vi "matrix_transpose_empty.vi"   [LabVIEW 2020]
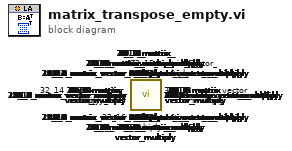
[diagram p0: block diagram]
diagram:
  n1 = call <vilib>:"32_16_matrix_vector_multiply.vi"() -> ()  [unwired: 6 in, 1 out]
  n2 = call <vilib>:"32_15_matrix_vector_multiply.vi"() -> ()  [unwired: 6 in, 1 out]
  n3 = call <vilib>:"32_14_matrix_vector_multiply.vi"() -> ()  [unwired: 6 in, 1 out]
  n4 = call <vilib>:"32_13_matrix_vector_multiply.vi"() -> ()  [unwired: 6 in, 1 out]
  n5 = call <vilib>:"32_12_matrix_vector_multiply.vi"() -> ()  [unwired: 6 in, 1 out]
  n6 = call <vilib>:"32_11_matrix_vector_multiply.vi"() -> ()  [unwired: 6 in, 1 out]
  n7 = call <vilib>:"32_10_matrix_vector_multiply.vi"() -> ()  [unwired: 6 in, 1 out]
  n8 = call <vilib>:"32_9_matrix_vector_multiply.vi"() -> ()  [unwired: 6 in, 1 out]
  n9 = call <vilib>:"32_8_matrix_vector_multiply.vi"() -> ()  [unwired: 6 in, 1 out]
  n10 = call <vilib>:"32_7_matrix_vector_multiply.vi"() -> ()  [unwired: 6 in, 1 out]
  n11 = call <vilib>:"32_6_matrix_vector_multiply.vi"() -> ()  [unwired: 6 in, 1 out]
  n12 = call <vilib>:"32_5_matrix_vector_multiply.vi"() -> ()  [unwired: 6 in, 1 out]
  n13 = call <vilib>:"32_4_matrix_vector_multiply.vi"() -> ()  [unwired: 6 in, 1 out]
  n14 = call <vilib>:"32_3_matrix_vector_multiply.vi"() -> ()  [unwired: 6 in, 1 out]
  n15 = call <vilib>:"32_2_matrix_vector_multiply.vi"() -> ()  [unwired: 6 in, 1 out]
  n16 = call <vilib>:"32_1_matrix_vector_multiply.vi"() -> ()  [unwired: 6 in, 1 out]
  n17 = call <vilib>:"31_16_matrix_vector_multiply.vi"() -> ()  [unwired: 6 in, 1 out]
  n18 = call <vilib>:"31_15_matrix_vector_multiply.vi"() -> ()  [unwired: 6 in, 1 out]
  n19 = call <vilib>:"31_14_matrix_vector_multiply.vi"() -> ()  [unwired: 6 in, 1 out]
  n20 = call <vilib>:"31_13_matrix_vector_multiply.vi"() -> ()  [unwired: 6 in, 1 out]
  n21 = call <vilib>:"31_12_matrix_vector_multiply.vi"() -> ()  [unwired: 6 in, 1 out]
  n22 = call <vilib>:"31_11_matrix_vector_multiply.vi"() -> ()  [unwired: 6 in, 1 out]
  n23 = call <vilib>:"31_10_matrix_vector_multiply.vi"() -> ()  [unwired: 6 in, 1 out]
  n24 = call <vilib>:"31_9_matrix_vector_multiply.vi"() -> ()  [unwired: 6 in, 1 out]
  n25 = call <vilib>:"31_8_matrix_vector_multiply.vi"() -> ()  [unwired: 6 in, 1 out]
  n26 = call <vilib>:"31_7_matrix_vector_multiply.vi"() -> ()  [unwired: 6 in, 1 out]
  n27 = call <vilib>:"31_6_matrix_vector_multiply.vi"() -> ()  [unwired: 6 in, 1 out]
  n28 = call <vilib>:"31_5_matrix_vector_multiply.vi"() -> ()  [unwired: 6 in, 1 out]
  n29 = call <vilib>:"31_4_matrix_vector_multiply.vi"() -> ()  [unwired: 6 in, 1 out]
  n30 = call <vilib>:"31_3_matrix_vector_multiply.vi"() -> ()  [unwired: 6 in, 1 out]
  n31 = call <vilib>:"31_2_matrix_vector_multiply.vi"() -> ()  [unwired: 6 in, 1 out]
  n32 = call <vilib>:"31_1_matrix_vector_multiply.vi"() -> ()  [unwired: 6 in, 1 out]
  n33 = call <vilib>:"30_16_matrix_vector_multiply.vi"() -> ()  [unwired: 6 in, 1 out]
  n34 = call <vilib>:"30_15_matrix_vector_multiply.vi"() -> ()  [unwired: 6 in, 1 out]
  n35 = call <vilib>:"30_14_matrix_vector_multiply.vi"() -> ()  [unwired: 6 in, 1 out]
  n36 = call <vilib>:"30_13_matrix_vector_multiply.vi"() -> ()  [unwired: 6 in, 1 out]
  n37 = call <vilib>:"30_12_matrix_vector_multiply.vi"() -> ()  [unwired: 6 in, 1 out]
  n38 = call <vilib>:"30_11_matrix_vector_multiply.vi"() -> ()  [unwired: 6 in, 1 out]
  n39 = call <vilib>:"30_10_matrix_vector_multiply.vi"() -> ()  [unwired: 6 in, 1 out]
  n40 = call <vilib>:"30_9_matrix_vector_multiply.vi"() -> ()  [unwired: 6 in, 1 out]
  n41 = call <vilib>:"30_8_matrix_vector_multiply.vi"() -> ()  [unwired: 6 in, 1 out]
  n42 = call <vilib>:"30_7_matrix_vector_multiply.vi"() -> ()  [unwired: 6 in, 1 out]
  n43 = call <vilib>:"30_6_matrix_vector_multiply.vi"() -> ()  [unwired: 6 in, 1 out]
  n44 = call <vilib>:"30_5_matrix_vector_multiply.vi"() -> ()  [unwired: 6 in, 1 out]
  n45 = call <vilib>:"30_4_matrix_vector_multiply.vi"() -> ()  [unwired: 6 in, 1 out]
  n46 = call <vilib>:"30_3_matrix_vector_multiply.vi"() -> ()  [unwired: 6 in, 1 out]
  n47 = call <vilib>:"30_2_matrix_vector_multiply.vi"() -> ()  [unwired: 6 in, 1 out]
  n48 = call <vilib>:"30_1_matrix_vector_multiply.vi"() -> ()  [unwired: 6 in, 1 out]
  n49 = call <vilib>:"29_16_matrix_vector_multiply.vi"() -> ()  [unwired: 6 in, 1 out]
  n50 = call <vilib>:"29_15_matrix_vector_multiply.vi"() -> ()  [unwired: 6 in, 1 out]
  n51 = call <vilib>:"29_14_matrix_vector_multiply.vi"() -> ()  [unwired: 6 in, 1 out]
  n52 = call <vilib>:"29_13_matrix_vector_multiply.vi"() -> ()  [unwired: 6 in, 1 out]
  n53 = call <vilib>:"29_12_matrix_vector_multiply.vi"() -> ()  [unwired: 6 in, 1 out]
  n54 = call <vilib>:"29_11_matrix_vector_multiply.vi"() -> ()  [unwired: 6 in, 1 out]
  n55 = call <vilib>:"29_10_matrix_vector_multiply.vi"() -> ()  [unwired: 6 in, 1 out]
  n56 = call <vilib>:"29_9_matrix_vector_multiply.vi"() -> ()  [unwired: 6 in, 1 out]
  n57 = call <vilib>:"29_8_matrix_vector_multiply.vi"() -> ()  [unwired: 6 in, 1 out]
  n58 = call <vilib>:"29_7_matrix_vector_multiply.vi"() -> ()  [unwired: 6 in, 1 out]
  n59 = call <vilib>:"29_6_matrix_vector_multiply.vi"() -> ()  [unwired: 6 in, 1 out]
  n60 = call <vilib>:"29_5_matrix_vector_multiply.vi"() -> ()  [unwired: 6 in, 1 out]
  n61 = call <vilib>:"29_4_matrix_vector_multiply.vi"() -> ()  [unwired: 6 in, 1 out]
  n62 = call <vilib>:"29_3_matrix_vector_multiply.vi"() -> ()  [unwired: 6 in, 1 out]
  n63 = call <vilib>:"29_2_matrix_vector_multiply.vi"() -> ()  [unwired: 6 in, 1 out]
  n64 = call <vilib>:"29_1_matrix_vector_multiply.vi"() -> ()  [unwired: 6 in, 1 out]
  n65 = call <vilib>:"28_16_matrix_vector_multiply.vi"() -> ()  [unwired: 6 in, 1 out]
  n66 = call <vilib>:"28_15_matrix_vector_multiply.vi"() -> ()  [unwired: 6 in, 1 out]
  n67 = call <vilib>:"28_14_matrix_vector_multiply.vi"() -> ()  [unwired: 6 in, 1 out]
  n68 = call <vilib>:"28_13_matrix_vector_multiply.vi"() -> ()  [unwired: 6 in, 1 out]
  n69 = call <vilib>:"28_12_matrix_vector_multiply.vi"() -> ()  [unwired: 6 in, 1 out]
  n70 = call <vilib>:"28_11_matrix_vector_multiply.vi"() -> ()  [unwired: 6 in, 1 out]
  n71 = call <vilib>:"28_10_matrix_vector_multiply.vi"() -> ()  [unwired: 6 in, 1 out]
  n72 = call <vilib>:"28_9_matrix_vector_multiply.vi"() -> ()  [unwired: 6 in, 1 out]
  n73 = call <vilib>:"28_8_matrix_vector_multiply.vi"() -> ()  [unwired: 6 in, 1 out]
  n74 = call <vilib>:"28_7_matrix_vector_multiply.vi"() -> ()  [unwired: 6 in, 1 out]
  n75 = call <vilib>:"28_6_matrix_vector_multiply.vi"() -> ()  [unwired: 6 in, 1 out]
  n76 = call <vilib>:"28_5_matrix_vector_multiply.vi"() -> ()  [unwired: 6 in, 1 out]
  n77 = call <vilib>:"28_4_matrix_vector_multiply.vi"() -> ()  [unwired: 6 in, 1 out]
  n78 = call <vilib>:"28_3_matrix_vector_multiply.vi"() -> ()  [unwired: 6 in, 1 out]
  n79 = call <vilib>:"28_2_matrix_vector_multiply.vi"() -> ()  [unwired: 6 in, 1 out]
  n80 = call <vilib>:"28_1_matrix_vector_multiply.vi"() -> ()  [unwired: 6 in, 1 out]
  n81 = call <vilib>:"27_16_matrix_vector_multiply.vi"() -> ()  [unwired: 6 in, 1 out]
  n82 = call <vilib>:"27_15_matrix_vector_multiply.vi"() -> ()  [unwired: 6 in, 1 out]
  n83 = call <vilib>:"27_14_matrix_vector_multiply.vi"() -> ()  [unwired: 6 in, 1 out]
  n84 = call <vilib>:"27_13_matrix_vector_multiply.vi"() -> ()  [unwired: 6 in, 1 out]
  n85 = call <vilib>:"27_12_matrix_vector_multiply.vi"() -> ()  [unwired: 6 in, 1 out]
  n86 = call <vilib>:"27_11_matrix_vector_multiply.vi"() -> ()  [unwired: 6 in, 1 out]
  n87 = call <vilib>:"27_10_matrix_vector_multiply.vi"() -> ()  [unwired: 6 in, 1 out]
  n88 = call <vilib>:"27_9_matrix_vector_multiply.vi"() -> ()  [unwired: 6 in, 1 out]
  n89 = call <vilib>:"27_8_matrix_vector_multiply.vi"() -> ()  [unwired: 6 in, 1 out]
  n90 = call <vilib>:"27_7_matrix_vector_multiply.vi"() -> ()  [unwired: 6 in, 1 out]
  n91 = call <vilib>:"27_6_matrix_vector_multiply.vi"() -> ()  [unwired: 6 in, 1 out]
  n92 = call <vilib>:"27_5_matrix_vector_multiply.vi"() -> ()  [unwired: 6 in, 1 out]
  n93 = call <vilib>:"27_4_matrix_vector_multiply.vi"() -> ()  [unwired: 6 in, 1 out]
  n94 = call <vilib>:"27_3_matrix_vector_multiply.vi"() -> ()  [unwired: 6 in, 1 out]
  n95 = call <vilib>:"27_2_matrix_vector_multiply.vi"() -> ()  [unwired: 6 in, 1 out]
  n96 = call <vilib>:"27_1_matrix_vector_multiply.vi"() -> ()  [unwired: 6 in, 1 out]
  n97 = call <vilib>:"26_16_matrix_vector_multiply.vi"() -> ()  [unwired: 6 in, 1 out]
  n98 = call <vilib>:"26_15_matrix_vector_multiply.vi"() -> ()  [unwired: 6 in, 1 out]
  n99 = call <vilib>:"26_14_matrix_vector_multiply.vi"() -> ()  [unwired: 6 in, 1 out]
  n100 = call <vilib>:"26_13_matrix_vector_multiply.vi"() -> ()  [unwired: 6 in, 1 out]
  n101 = call <vilib>:"26_12_matrix_vector_multiply.vi"() -> ()  [unwired: 6 in, 1 out]
  n102 = call <vilib>:"26_11_matrix_vector_multiply.vi"() -> ()  [unwired: 6 in, 1 out]
  n103 = call <vilib>:"26_10_matrix_vector_multiply.vi"() -> ()  [unwired: 6 in, 1 out]
  n104 = call <vilib>:"26_9_matrix_vector_multiply.vi"() -> ()  [unwired: 6 in, 1 out]
  n105 = call <vilib>:"26_8_matrix_vector_multiply.vi"() -> ()  [unwired: 6 in, 1 out]
  n106 = call <vilib>:"26_7_matrix_vector_multiply.vi"() -> ()  [unwired: 6 in, 1 out]
  n107 = call <vilib>:"26_6_matrix_vector_multiply.vi"() -> ()  [unwired: 6 in, 1 out]
  n108 = call <vilib>:"26_5_matrix_vector_multiply.vi"() -> ()  [unwired: 6 in, 1 out]
  n109 = call <vilib>:"26_4_matrix_vector_multiply.vi"() -> ()  [unwired: 6 in, 1 out]
  n110 = call <vilib>:"26_3_matrix_vector_multiply.vi"() -> ()  [unwired: 6 in, 1 out]
  n111 = call <vilib>:"26_2_matrix_vector_multiply.vi"() -> ()  [unwired: 6 in, 1 out]
  n112 = call <vilib>:"26_1_matrix_vector_multiply.vi"() -> ()  [unwired: 6 in, 1 out]
  n113 = call <vilib>:"25_16_matrix_vector_multiply.vi"() -> ()  [unwired: 6 in, 1 out]
  n114 = call <vilib>:"25_15_matrix_vector_multiply.vi"() -> ()  [unwired: 6 in, 1 out]
  n115 = call <vilib>:"25_14_matrix_vector_multiply.vi"() -> ()  [unwired: 6 in, 1 out]
  n116 = call <vilib>:"25_13_matrix_vector_multiply.vi"() -> ()  [unwired: 6 in, 1 out]
  n117 = call <vilib>:"25_12_matrix_vector_multiply.vi"() -> ()  [unwired: 6 in, 1 out]
  n118 = call <vilib>:"25_11_matrix_vector_multiply.vi"() -> ()  [unwired: 6 in, 1 out]
  n119 = call <vilib>:"25_10_matrix_vector_multiply.vi"() -> ()  [unwired: 6 in, 1 out]
  n120 = call <vilib>:"25_9_matrix_vector_multiply.vi"() -> ()  [unwired: 6 in, 1 out]
  n121 = call <vilib>:"25_8_matrix_vector_multiply.vi"() -> ()  [unwired: 6 in, 1 out]
  n122 = call <vilib>:"25_7_matrix_vector_multiply.vi"() -> ()  [unwired: 6 in, 1 out]
  n123 = call <vilib>:"25_6_matrix_vector_multiply.vi"() -> ()  [unwired: 6 in, 1 out]
  n124 = call <vilib>:"25_5_matrix_vector_multiply.vi"() -> ()  [unwired: 6 in, 1 out]
  n125 = call <vilib>:"25_4_matrix_vector_multiply.vi"() -> ()  [unwired: 6 in, 1 out]
  n126 = call <vilib>:"25_3_matrix_vector_multiply.vi"() -> ()  [unwired: 6 in, 1 out]
  n127 = call <vilib>:"25_2_matrix_vector_multiply.vi"() -> ()  [unwired: 6 in, 1 out]
  n128 = call <vilib>:"25_1_matrix_vector_multiply.vi"() -> ()  [unwired: 6 in, 1 out]
  n129 = call <vilib>:"24_16_matrix_vector_multiply.vi"() -> ()  [unwired: 6 in, 1 out]
  n130 = call <vilib>:"24_15_matrix_vector_multiply.vi"() -> ()  [unwired: 6 in, 1 out]
  n131 = call <vilib>:"24_14_matrix_vector_multiply.vi"() -> ()  [unwired: 6 in, 1 out]
  n132 = call <vilib>:"24_13_matrix_vector_multiply.vi"() -> ()  [unwired: 6 in, 1 out]
  n133 = call <vilib>:"24_12_matrix_vector_multiply.vi"() -> ()  [unwired: 6 in, 1 out]
  n134 = call <vilib>:"24_11_matrix_vector_multiply.vi"() -> ()  [unwired: 6 in, 1 out]
  n135 = call <vilib>:"24_10_matrix_vector_multiply.vi"() -> ()  [unwired: 6 in, 1 out]
  n136 = call <vilib>:"24_9_matrix_vector_multiply.vi"() -> ()  [unwired: 6 in, 1 out]
  n137 = call <vilib>:"24_8_matrix_vector_multiply.vi"() -> ()  [unwired: 6 in, 1 out]
  n138 = call <vilib>:"24_7_matrix_vector_multiply.vi"() -> ()  [unwired: 6 in, 1 out]
  n139 = call <vilib>:"24_6_matrix_vector_multiply.vi"() -> ()  [unwired: 6 in, 1 out]
  n140 = call <vilib>:"24_5_matrix_vector_multiply.vi"() -> ()  [unwired: 6 in, 1 out]
  n141 = call <vilib>:"24_4_matrix_vector_multiply.vi"() -> ()  [unwired: 6 in, 1 out]
  n142 = call <vilib>:"24_3_matrix_vector_multiply.vi"() -> ()  [unwired: 6 in, 1 out]
  n143 = call <vilib>:"24_2_matrix_vector_multiply.vi"() -> ()  [unwired: 6 in, 1 out]
  n144 = call <vilib>:"24_1_matrix_vector_multiply.vi"() -> ()  [unwired: 6 in, 1 out]
  n145 = call <vilib>:"23_16_matrix_vector_multiply.vi"() -> ()  [unwired: 6 in, 1 out]
  n146 = call <vilib>:"23_15_matrix_vector_multiply.vi"() -> ()  [unwired: 6 in, 1 out]
  n147 = call <vilib>:"23_14_matrix_vector_multiply.vi"() -> ()  [unwired: 6 in, 1 out]
  n148 = call <vilib>:"23_13_matrix_vector_multiply.vi"() -> ()  [unwired: 6 in, 1 out]
  n149 = call <vilib>:"23_12_matrix_vector_multiply.vi"() -> ()  [unwired: 6 in, 1 out]
  n150 = call <vilib>:"23_11_matrix_vector_multiply.vi"() -> ()  [unwired: 6 in, 1 out]
  n151 = call <vilib>:"23_10_matrix_vector_multiply.vi"() -> ()  [unwired: 6 in, 1 out]
  n152 = call <vilib>:"23_9_matrix_vector_multiply.vi"() -> ()  [unwired: 6 in, 1 out]
  n153 = call <vilib>:"23_8_matrix_vector_multiply.vi"() -> ()  [unwired: 6 in, 1 out]
  n154 = call <vilib>:"23_7_matrix_vector_multiply.vi"() -> ()  [unwired: 6 in, 1 out]
  n155 = call <vilib>:"23_6_matrix_vector_multiply.vi"() -> ()  [unwired: 6 in, 1 out]
  n156 = call <vilib>:"23_5_matrix_vector_multiply.vi"() -> ()  [unwired: 6 in, 1 out]
  n157 = call <vilib>:"23_4_matrix_vector_multiply.vi"() -> ()  [unwired: 6 in, 1 out]
  n158 = call <vilib>:"23_3_matrix_vector_multiply.vi"() -> ()  [unwired: 6 in, 1 out]
  n159 = call <vilib>:"23_2_matrix_vector_multiply.vi"() -> ()  [unwired: 6 in, 1 out]
  n160 = call <vilib>:"23_1_matrix_vector_multiply.vi"() -> ()  [unwired: 6 in, 1 out]
  n161 = call <vilib>:"22_16_matrix_vector_multiply.vi"() -> ()  [unwired: 6 in, 1 out]
  n162 = call <vilib>:"22_15_matrix_vector_multiply.vi"() -> ()  [unwired: 6 in, 1 out]
  n163 = call <vilib>:"22_14_matrix_vector_multiply.vi"() -> ()  [unwired: 6 in, 1 out]
  n164 = call <vilib>:"22_13_matrix_vector_multiply.vi"() -> ()  [unwired: 6 in, 1 out]
  n165 = call <vilib>:"22_12_matrix_vector_multiply.vi"() -> ()  [unwired: 6 in, 1 out]
  n166 = call <vilib>:"22_11_matrix_vector_multiply.vi"() -> ()  [unwired: 6 in, 1 out]
  n167 = call <vilib>:"22_10_matrix_vector_multiply.vi"() -> ()  [unwired: 6 in, 1 out]
  n168 = call <vilib>:"22_9_matrix_vector_multiply.vi"() -> ()  [unwired: 6 in, 1 out]
  n169 = call <vilib>:"22_8_matrix_vector_multiply.vi"() -> ()  [unwired: 6 in, 1 out]
  n170 = call <vilib>:"22_7_matrix_vector_multiply.vi"() -> ()  [unwired: 6 in, 1 out]
  n171 = call <vilib>:"22_6_matrix_vector_multiply.vi"() -> ()  [unwired: 6 in, 1 out]
  n172 = call <vilib>:"22_5_matrix_vector_multiply.vi"() -> ()  [unwired: 6 in, 1 out]
  n173 = call <vilib>:"22_4_matrix_vector_multiply.vi"() -> ()  [unwired: 6 in, 1 out]
  n174 = call <vilib>:"22_3_matrix_vector_multiply.vi"() -> ()  [unwired: 6 in, 1 out]
  n175 = call <vilib>:"22_2_matrix_vector_multiply.vi"() -> ()  [unwired: 6 in, 1 out]
  n176 = call <vilib>:"22_1_matrix_vector_multiply.vi"() -> ()  [unwired: 6 in, 1 out]
  n177 = call <vilib>:"21_16_matrix_vector_multiply.vi"() -> ()  [unwired: 6 in, 1 out]
  n178 = call <vilib>:"21_15_matrix_vector_multiply.vi"() -> ()  [unwired: 6 in, 1 out]
  n179 = call <vilib>:"21_14_matrix_vector_multiply.vi"() -> ()  [unwired: 6 in, 1 out]
  n180 = call <vilib>:"21_13_matrix_vector_multiply.vi"() -> ()  [unwired: 6 in, 1 out]
  n181 = call <vilib>:"21_12_matrix_vector_multiply.vi"() -> ()  [unwired: 6 in, 1 out]
  n182 = call <vilib>:"21_11_matrix_vector_multiply.vi"() -> ()  [unwired: 6 in, 1 out]
  n183 = call <vilib>:"21_10_matrix_vector_multiply.vi"() -> ()  [unwired: 6 in, 1 out]
  n184 = call <vilib>:"21_9_matrix_vector_multiply.vi"() -> ()  [unwired: 6 in, 1 out]
  n185 = call <vilib>:"21_8_matrix_vector_multiply.vi"() -> ()  [unwired: 6 in, 1 out]
  n186 = call <vilib>:"21_7_matrix_vector_multiply.vi"() -> ()  [unwired: 6 in, 1 out]
  n187 = call <vilib>:"21_6_matrix_vector_multiply.vi"() -> ()  [unwired: 6 in, 1 out]
  n188 = call <vilib>:"21_5_matrix_vector_multiply.vi"() -> ()  [unwired: 6 in, 1 out]
  n189 = call <vilib>:"21_4_matrix_vector_multiply.vi"() -> ()  [unwired: 6 in, 1 out]
  n190 = call <vilib>:"21_3_matrix_vector_multiply.vi"() -> ()  [unwired: 6 in, 1 out]
  n191 = call <vilib>:"21_2_matrix_vector_multiply.vi"() -> ()  [unwired: 6 in, 1 out]
  n192 = call <vilib>:"21_1_matrix_vector_multiply.vi"() -> ()  [unwired: 6 in, 1 out]
  n193 = call <vilib>:"20_16_matrix_vector_multiply.vi"() -> ()  [unwired: 6 in, 1 out]
  n194 = call <vilib>:"20_15_matrix_vector_multiply.vi"() -> ()  [unwired: 6 in, 1 out]
  n195 = call <vilib>:"20_14_matrix_vector_multiply.vi"() -> ()  [unwired: 6 in, 1 out]
  n196 = call <vilib>:"20_13_matrix_vector_multiply.vi"() -> ()  [unwired: 6 in, 1 out]
  n197 = call <vilib>:"20_12_matrix_vector_multiply.vi"() -> ()  [unwired: 6 in, 1 out]
  n198 = call <vilib>:"20_11_matrix_vector_multiply.vi"() -> ()  [unwired: 6 in, 1 out]
  n199 = call <vilib>:"20_10_matrix_vector_multiply.vi"() -> ()  [unwired: 6 in, 1 out]
  n200 = call <vilib>:"20_9_matrix_vector_multiply.vi"() -> ()  [unwired: 6 in, 1 out]
  n201 = call <vilib>:"20_8_matrix_vector_multiply.vi"() -> ()  [unwired: 6 in, 1 out]
  n202 = call <vilib>:"20_7_matrix_vector_multiply.vi"() -> ()  [unwired: 6 in, 1 out]
  n203 = call <vilib>:"20_6_matrix_vector_multiply.vi"() -> ()  [unwired: 6 in, 1 out]
  n204 = call <vilib>:"20_5_matrix_vector_multiply.vi"() -> ()  [unwired: 6 in, 1 out]
  n205 = call <vilib>:"20_4_matrix_vector_multiply.vi"() -> ()  [unwired: 6 in, 1 out]
  n206 = call <vilib>:"20_3_matrix_vector_multiply.vi"() -> ()  [unwired: 6 in, 1 out]
  n207 = call <vilib>:"20_2_matrix_vector_multiply.vi"() -> ()  [unwired: 6 in, 1 out]
  n208 = call <vilib>:"20_1_matrix_vector_multiply.vi"() -> ()  [unwired: 6 in, 1 out]
  n209 = call <vilib>:"19_16_matrix_vector_multiply.vi"() -> ()  [unwired: 6 in, 1 out]
  n210 = call <vilib>:"19_15_matrix_vector_multiply.vi"() -> ()  [unwired: 6 in, 1 out]
  n211 = call <vilib>:"19_14_matrix_vector_multiply.vi"() -> ()  [unwired: 6 in, 1 out]
  n212 = call <vilib>:"19_13_matrix_vector_multiply.vi"() -> ()  [unwired: 6 in, 1 out]
  n213 = call <vilib>:"19_12_matrix_vector_multiply.vi"() -> ()  [unwired: 6 in, 1 out]
  n214 = call <vilib>:"19_11_matrix_vector_multiply.vi"() -> ()  [unwired: 6 in, 1 out]
  n215 = call <vilib>:"19_10_matrix_vector_multiply.vi"() -> ()  [unwired: 6 in, 1 out]
  n216 = call <vilib>:"19_9_matrix_vector_multiply.vi"() -> ()  [unwired: 6 in, 1 out]
  n217 = call <vilib>:"19_8_matrix_vector_multiply.vi"() -> ()  [unwired: 6 in, 1 out]
  n218 = call <vilib>:"19_7_matrix_vector_multiply.vi"() -> ()  [unwired: 6 in, 1 out]
  n219 = call <vilib>:"19_6_matrix_vector_multiply.vi"() -> ()  [unwired: 6 in, 1 out]
  n220 = call <vilib>:"19_5_matrix_vector_multiply.vi"() -> ()  [unwired: 6 in, 1 out]
  n221 = call <vilib>:"19_4_matrix_vector_multiply.vi"() -> ()  [unwired: 6 in, 1 out]
  n222 = call <vilib>:"19_3_matrix_vector_multiply.vi"() -> ()  [unwired: 6 in, 1 out]
  n223 = call <vilib>:"19_2_matrix_vector_multiply.vi"() -> ()  [unwired: 6 in, 1 out]
  n224 = call <vilib>:"19_1_matrix_vector_multiply.vi"() -> ()  [unwired: 6 in, 1 out]
  n225 = call <vilib>:"18_16_matrix_vector_multiply.vi"() -> ()  [unwired: 6 in, 1 out]
  n226 = call <vilib>:"18_15_matrix_vector_multiply.vi"() -> ()  [unwired: 6 in, 1 out]
  n227 = call <vilib>:"18_14_matrix_vector_multiply.vi"() -> ()  [unwired: 6 in, 1 out]
  n228 = call <vilib>:"18_13_matrix_vector_multiply.vi"() -> ()  [unwired: 6 in, 1 out]
  n229 = call <vilib>:"18_12_matrix_vector_multiply.vi"() -> ()  [unwired: 6 in, 1 out]
  n230 = call <vilib>:"18_11_matrix_vector_multiply.vi"() -> ()  [unwired: 6 in, 1 out]
  n231 = call <vilib>:"18_10_matrix_vector_multiply.vi"() -> ()  [unwired: 6 in, 1 out]
  n232 = call <vilib>:"18_9_matrix_vector_multiply.vi"() -> ()  [unwired: 6 in, 1 out]
  n233 = call <vilib>:"18_8_matrix_vector_multiply.vi"() -> ()  [unwired: 6 in, 1 out]
  n234 = call <vilib>:"18_7_matrix_vector_multiply.vi"() -> ()  [unwired: 6 in, 1 out]
  n235 = call <vilib>:"18_6_matrix_vector_multiply.vi"() -> ()  [unwired: 6 in, 1 out]
  n236 = call <vilib>:"18_5_matrix_vector_multiply.vi"() -> ()  [unwired: 6 in, 1 out]
  n237 = call <vilib>:"18_4_matrix_vector_multiply.vi"() -> ()  [unwired: 6 in, 1 out]
  n238 = call <vilib>:"18_3_matrix_vector_multiply.vi"() -> ()  [unwired: 6 in, 1 out]
  n239 = call <vilib>:"18_2_matrix_vector_multiply.vi"() -> ()  [unwired: 6 in, 1 out]
  n240 = call <vilib>:"18_1_matrix_vector_multiply.vi"() -> ()  [unwired: 6 in, 1 out]
  n241 = call <vilib>:"17_16_matrix_vector_multiply.vi"() -> ()  [unwired: 6 in, 1 out]
  n242 = call <vilib>:"17_15_matrix_vector_multiply.vi"() -> ()  [unwired: 6 in, 1 out]
  n243 = call <vilib>:"17_14_matrix_vector_multiply.vi"() -> ()  [unwired: 6 in, 1 out]
  n244 = call <vilib>:"17_13_matrix_vector_multiply.vi"() -> ()  [unwired: 6 in, 1 out]
  n245 = call <vilib>:"17_12_matrix_vector_multiply.vi"() -> ()  [unwired: 6 in, 1 out]
  n246 = call <vilib>:"17_11_matrix_vector_multiply.vi"() -> ()  [unwired: 6 in, 1 out]
  n247 = call <vilib>:"17_10_matrix_vector_multiply.vi"() -> ()  [unwired: 6 in, 1 out]
  n248 = call <vilib>:"17_9_matrix_vector_multiply.vi"() -> ()  [unwired: 6 in, 1 out]
  n249 = call <vilib>:"17_8_matrix_vector_multiply.vi"() -> ()  [unwired: 6 in, 1 out]
  n250 = call <vilib>:"17_7_matrix_vector_multiply.vi"() -> ()  [unwired: 6 in, 1 out]
  n251 = call <vilib>:"17_6_matrix_vector_multiply.vi"() -> ()  [unwired: 6 in, 1 out]
  n252 = call <vilib>:"17_5_matrix_vector_multiply.vi"() -> ()  [unwired: 6 in, 1 out]
  n253 = call <vilib>:"17_4_matrix_vector_multiply.vi"() -> ()  [unwired: 6 in, 1 out]
  n254 = call <vilib>:"17_3_matrix_vector_multiply.vi"() -> ()  [unwired: 6 in, 1 out]
  n255 = call <vilib>:"17_2_matrix_vector_multiply.vi"() -> ()  [unwired: 6 in, 1 out]
  n256 = call <vilib>:"17_1_matrix_vector_multiply.vi"() -> ()  [unwired: 6 in, 1 out]
  n257 = call <vilib>:"16_16_matrix_vector_multiply.vi"() -> ()  [unwired: 6 in, 1 out]
  n258 = call <vilib>:"16_15_matrix_vector_multiply.vi"() -> ()  [unwired: 6 in, 1 out]
  n259 = call <vilib>:"16_14_matrix_vector_multiply.vi"() -> ()  [unwired: 6 in, 1 out]
  n260 = call <vilib>:"16_13_matrix_vector_multiply.vi"() -> ()  [unwired: 6 in, 1 out]
  n261 = call <vilib>:"16_12_matrix_vector_multiply.vi"() -> ()  [unwired: 6 in, 1 out]
  n262 = call <vilib>:"16_11_matrix_vector_multiply.vi"() -> ()  [unwired: 6 in, 1 out]
  n263 = call <vilib>:"16_10_matrix_vector_multiply.vi"() -> ()  [unwired: 6 in, 1 out]
  n264 = call <vilib>:"16_9_matrix_vector_multiply.vi"() -> ()  [unwired: 6 in, 1 out]
  n265 = call <vilib>:"16_8_matrix_vector_multiply.vi"() -> ()  [unwired: 6 in, 1 out]
  n266 = call <vilib>:"16_7_matrix_vector_multiply.vi"() -> ()  [unwired: 6 in, 1 out]
  n267 = call <vilib>:"16_6_matrix_vector_multiply.vi"() -> ()  [unwired: 6 in, 1 out]
  n268 = call <vilib>:"16_5_matrix_vector_multiply.vi"() -> ()  [unwired: 6 in, 1 out]
  n269 = call <vilib>:"16_4_matrix_vector_multiply.vi"() -> ()  [unwired: 6 in, 1 out]
  n270 = call <vilib>:"16_3_matrix_vector_multiply.vi"() -> ()  [unwired: 6 in, 1 out]
  n271 = call <vilib>:"16_2_matrix_vector_multiply.vi"() -> ()  [unwired: 6 in, 1 out]
  n272 = call <vilib>:"16_1_matrix_vector_multiply.vi"() -> ()  [unwired: 6 in, 1 out]
  n273 = call <vilib>:"15_16_matrix_vector_multiply.vi"() -> ()  [unwired: 6 in, 1 out]
  n274 = call <vilib>:"15_15_matrix_vector_multiply.vi"() -> ()  [unwired: 6 in, 1 out]
  n275 = call <vilib>:"15_14_matrix_vector_multiply.vi"() -> ()  [unwired: 6 in, 1 out]
  n276 = call <vilib>:"15_13_matrix_vector_multiply.vi"() -> ()  [unwired: 6 in, 1 out]
  n277 = call <vilib>:"15_12_matrix_vector_multiply.vi"() -> ()  [unwired: 6 in, 1 out]
  n278 = call <vilib>:"15_11_matrix_vector_multiply.vi"() -> ()  [unwired: 6 in, 1 out]
  n279 = call <vilib>:"15_10_matrix_vector_multiply.vi"() -> ()  [unwired: 6 in, 1 out]
  n280 = call <vilib>:"15_9_matrix_vector_multiply.vi"() -> ()  [unwired: 6 in, 1 out]
  n281 = call <vilib>:"15_8_matrix_vector_multiply.vi"() -> ()  [unwired: 6 in, 1 out]
  n282 = call <vilib>:"15_7_matrix_vector_multiply.vi"() -> ()  [unwired: 6 in, 1 out]
  n283 = call <vilib>:"15_6_matrix_vector_multiply.vi"() -> ()  [unwired: 6 in, 1 out]
  n284 = call <vilib>:"15_5_matrix_vector_multiply.vi"() -> ()  [unwired: 6 in, 1 out]
  n285 = call <vilib>:"15_4_matrix_vector_multiply.vi"() -> ()  [unwired: 6 in, 1 out]
  n286 = call <vilib>:"15_3_matrix_vector_multiply.vi"() -> ()  [unwired: 6 in, 1 out]
  n287 = call <vilib>:"15_2_matrix_vector_multiply.vi"() -> ()  [unwired: 6 in, 1 out]
  n288 = call <vilib>:"15_1_matrix_vector_multiply.vi"() -> ()  [unwired: 6 in, 1 out]
  n289 = call <vilib>:"14_16_matrix_vector_multiply.vi"() -> ()  [unwired: 6 in, 1 out]
  n290 = call <vilib>:"14_15_matrix_vector_multiply.vi"() -> ()  [unwired: 6 in, 1 out]
  n291 = call <vilib>:"14_14_matrix_vector_multiply.vi"() -> ()  [unwired: 6 in, 1 out]
  n292 = call <vilib>:"14_13_matrix_vector_multiply.vi"() -> ()  [unwired: 6 in, 1 out]
  n293 = call <vilib>:"14_12_matrix_vector_multiply.vi"() -> ()  [unwired: 6 in, 1 out]
  n294 = call <vilib>:"14_11_matrix_vector_multiply.vi"() -> ()  [unwired: 6 in, 1 out]
  n295 = call <vilib>:"14_10_matrix_vector_multiply.vi"() -> ()  [unwired: 6 in, 1 out]
  n296 = call <vilib>:"14_9_matrix_vector_multiply.vi"() -> ()  [unwired: 6 in, 1 out]
  n297 = call <vilib>:"14_8_matrix_vector_multiply.vi"() -> ()  [unwired: 6 in, 1 out]
  n298 = call <vilib>:"14_7_matrix_vector_multiply.vi"() -> ()  [unwired: 6 in, 1 out]
  n299 = call <vilib>:"14_6_matrix_vector_multiply.vi"() -> ()  [unwired: 6 in, 1 out]
  n300 = call <vilib>:"14_5_matrix_vector_multiply.vi"() -> ()  [unwired: 6 in, 1 out]
  n301 = call <vilib>:"14_4_matrix_vector_multiply.vi"() -> ()  [unwired: 6 in, 1 out]
  n302 = call <vilib>:"14_3_matrix_vector_multiply.vi"() -> ()  [unwired: 6 in, 1 out]
  n303 = call <vilib>:"14_2_matrix_vector_multiply.vi"() -> ()  [unwired: 6 in, 1 out]
  n304 = call <vilib>:"14_1_matrix_vector_multiply.vi"() -> ()  [unwired: 6 in, 1 out]
  n305 = call <vilib>:"13_16_matrix_vector_multiply.vi"() -> ()  [unwired: 6 in, 1 out]
  n306 = call <vilib>:"13_15_matrix_vector_multiply.vi"() -> ()  [unwired: 6 in, 1 out]
  n307 = call <vilib>:"13_14_matrix_vector_multiply.vi"() -> ()  [unwired: 6 in, 1 out]
  n308 = call <vilib>:"13_13_matrix_vector_multiply.vi"() -> ()  [unwired: 6 in, 1 out]
  n309 = call <vilib>:"13_12_matrix_vector_multiply.vi"() -> ()  [unwired: 6 in, 1 out]
  n310 = call <vilib>:"13_11_matrix_vector_multiply.vi"() -> ()  [unwired: 6 in, 1 out]
  n311 = call <vilib>:"13_10_matrix_vector_multiply.vi"() -> ()  [unwired: 6 in, 1 out]
  n312 = call <vilib>:"13_9_matrix_vector_multiply.vi"() -> ()  [unwired: 6 in, 1 out]
  n313 = call <vilib>:"13_8_matrix_vector_multiply.vi"() -> ()  [unwired: 6 in, 1 out]
  n314 = call <vilib>:"13_7_matrix_vector_multiply.vi"() -> ()  [unwired: 6 in, 1 out]
  n315 = call <vilib>:"13_6_matrix_vector_multiply.vi"() -> ()  [unwired: 6 in, 1 out]
  n316 = call <vilib>:"13_5_matrix_vector_multiply.vi"() -> ()  [unwired: 6 in, 1 out]
  n317 = call <vilib>:"13_4_matrix_vector_multiply.vi"() -> ()  [unwired: 6 in, 1 out]
  n318 = call <vilib>:"13_3_matrix_vector_multiply.vi"() -> ()  [unwired: 6 in, 1 out]
  n319 = call <vilib>:"13_2_matrix_vector_multiply.vi"() -> ()  [unwired: 6 in, 1 out]
  n320 = call <vilib>:"13_1_matrix_vector_multiply.vi"() -> ()  [unwired: 6 in, 1 out]
  n321 = call <vilib>:"12_16_matrix_vector_multiply.vi"() -> ()  [unwired: 6 in, 1 out]
  n322 = call <vilib>:"12_15_matrix_vector_multiply.vi"() -> ()  [unwired: 6 in, 1 out]
  n323 = call <vilib>:"12_14_matrix_vector_multiply.vi"() -> ()  [unwired: 6 in, 1 out]
  n324 = call <vilib>:"12_13_matrix_vector_multiply.vi"() -> ()  [unwired: 6 in, 1 out]
  n325 = call <vilib>:"12_12_matrix_vector_multiply.vi"() -> ()  [unwired: 6 in, 1 out]
  n326 = call <vilib>:"12_11_matrix_vector_multiply.vi"() -> ()  [unwired: 6 in, 1 out]
  n327 = call <vilib>:"12_10_matrix_vector_multiply.vi"() -> ()  [unwired: 6 in, 1 out]
  n328 = call <vilib>:"12_9_matrix_vector_multiply.vi"() -> ()  [unwired: 6 in, 1 out]
  n329 = call <vilib>:"12_8_matrix_vector_multiply.vi"() -> ()  [unwired: 6 in, 1 out]
  n330 = call <vilib>:"12_7_matrix_vector_multiply.vi"() -> ()  [unwired: 6 in, 1 out]
  n331 = call <vilib>:"12_6_matrix_vector_multiply.vi"() -> ()  [unwired: 6 in, 1 out]
  n332 = call <vilib>:"12_5_matrix_vector_multiply.vi"() -> ()  [unwired: 6 in, 1 out]
  n333 = call <vilib>:"12_4_matrix_vector_multiply.vi"() -> ()  [unwired: 6 in, 1 out]
  n334 = call <vilib>:"12_3_matrix_vector_multiply.vi"() -> ()  [unwired: 6 in, 1 out]
  n335 = call <vilib>:"12_2_matrix_vector_multiply.vi"() -> ()  [unwired: 6 in, 1 out]
  n336 = call <vilib>:"12_1_matrix_vector_multiply.vi"() -> ()  [unwired: 6 in, 1 out]
  n337 = call <vilib>:"11_16_matrix_vector_multiply.vi"() -> ()  [unwired: 6 in, 1 out]
  n338 = call <vilib>:"11_15_matrix_vector_multiply.vi"() -> ()  [unwired: 6 in, 1 out]
  n339 = call <vilib>:"11_14_matrix_vector_multiply.vi"() -> ()  [unwired: 6 in, 1 out]
  n340 = call <vilib>:"11_13_matrix_vector_multiply.vi"() -> ()  [unwired: 6 in, 1 out]
  n341 = call <vilib>:"11_12_matrix_vector_multiply.vi"() -> ()  [unwired: 6 in, 1 out]
  n342 = call <vilib>:"11_11_matrix_vector_multiply.vi"() -> ()  [unwired: 6 in, 1 out]
  n343 = call <vilib>:"11_10_matrix_vector_multiply.vi"() -> ()  [unwired: 6 in, 1 out]
  n344 = call <vilib>:"11_9_matrix_vector_multiply.vi"() -> ()  [unwired: 6 in, 1 out]
  n345 = call <vilib>:"11_8_matrix_vector_multiply.vi"() -> ()  [unwired: 6 in, 1 out]
  n346 = call <vilib>:"11_7_matrix_vector_multiply.vi"() -> ()  [unwired: 6 in, 1 out]
  n347 = call <vilib>:"11_6_matrix_vector_multiply.vi"() -> ()  [unwired: 6 in, 1 out]
  n348 = call <vilib>:"11_5_matrix_vector_multiply.vi"() -> ()  [unwired: 6 in, 1 out]
  n349 = call <vilib>:"11_4_matrix_vector_multiply.vi"() -> ()  [unwired: 6 in, 1 out]
  n350 = call <vilib>:"11_3_matrix_vector_multiply.vi"() -> ()  [unwired: 6 in, 1 out]
  n351 = call <vilib>:"11_2_matrix_vector_multiply.vi"() -> ()  [unwired: 6 in, 1 out]
  n352 = call <vilib>:"11_1_matrix_vector_multiply.vi"() -> ()  [unwired: 6 in, 1 out]
  n353 = call <vilib>:"10_16_matrix_vector_multiply.vi"() -> ()  [unwired: 6 in, 1 out]
  n354 = call <vilib>:"10_15_matrix_vector_multiply.vi"() -> ()  [unwired: 6 in, 1 out]
  n355 = call <vilib>:"10_14_matrix_vector_multiply.vi"() -> ()  [unwired: 6 in, 1 out]
  n356 = call <vilib>:"10_13_matrix_vector_multiply.vi"() -> ()  [unwired: 6 in, 1 out]
  n357 = call <vilib>:"10_12_matrix_vector_multiply.vi"() -> ()  [unwired: 6 in, 1 out]
  n358 = call <vilib>:"10_11_matrix_vector_multiply.vi"() -> ()  [unwired: 6 in, 1 out]
  n359 = call <vilib>:"10_10_matrix_vector_multiply.vi"() -> ()  [unwired: 6 in, 1 out]
  n360 = call <vilib>:"10_9_matrix_vector_multiply.vi"() -> ()  [unwired: 6 in, 1 out]
  n361 = call <vilib>:"10_8_matrix_vector_multiply.vi"() -> ()  [unwired: 6 in, 1 out]
  n362 = call <vilib>:"10_7_matrix_vector_multiply.vi"() -> ()  [unwired: 6 in, 1 out]
  n363 = call <vilib>:"10_6_matrix_vector_multiply.vi"() -> ()  [unwired: 6 in, 1 out]
  n364 = call <vilib>:"10_5_matrix_vector_multiply.vi"() -> ()  [unwired: 6 in, 1 out]
  n365 = call <vilib>:"10_4_matrix_vector_multiply.vi"() -> ()  [unwired: 6 in, 1 out]
  n366 = call <vilib>:"10_3_matrix_vector_multiply.vi"() -> ()  [unwired: 6 in, 1 out]
  n367 = call <vilib>:"10_2_matrix_vector_multiply.vi"() -> ()  [unwired: 6 in, 1 out]
  n368 = call <vilib>:"10_1_matrix_vector_multiply.vi"() -> ()  [unwired: 6 in, 1 out]
  n369 = call <vilib>:"9_16_matrix_vector_multiply.vi"() -> ()  [unwired: 6 in, 1 out]
  n370 = call <vilib>:"9_15_matrix_vector_multiply.vi"() -> ()  [unwired: 6 in, 1 out]
  n371 = call <vilib>:"9_14_matrix_vector_multiply.vi"() -> ()  [unwired: 6 in, 1 out]
  n372 = call <vilib>:"9_13_matrix_vector_multiply.vi"() -> ()  [unwired: 6 in, 1 out]
  n373 = call <vilib>:"9_12_matrix_vector_multiply.vi"() -> ()  [unwired: 6 in, 1 out]
  n374 = call <vilib>:"9_11_matrix_vector_multiply.vi"() -> ()  [unwired: 6 in, 1 out]
  n375 = call <vilib>:"9_10_matrix_vector_multiply.vi"() -> ()  [unwired: 6 in, 1 out]
  n376 = call <vilib>:"9_9_matrix_vector_multiply.vi"() -> ()  [unwired: 6 in, 1 out]
  n377 = call <vilib>:"9_8_matrix_vector_multiply.vi"() -> ()  [unwired: 6 in, 1 out]
  n378 = call <vilib>:"9_7_matrix_vector_multiply.vi"() -> ()  [unwired: 6 in, 1 out]
  n379 = call <vilib>:"9_6_matrix_vector_multiply.vi"() -> ()  [unwired: 6 in, 1 out]
  n380 = call <vilib>:"9_5_matrix_vector_multiply.vi"() -> ()  [unwired: 6 in, 1 out]
  n381 = call <vilib>:"9_4_matrix_vector_multiply.vi"() -> ()  [unwired: 6 in, 1 out]
  n382 = call <vilib>:"9_3_matrix_vector_multiply.vi"() -> ()  [unwired: 6 in, 1 out]
  n383 = call <vilib>:"9_2_matrix_vector_multiply.vi"() -> ()  [unwired: 6 in, 1 out]
  n384 = call <vilib>:"9_1_matrix_vector_multiply.vi"() -> ()  [unwired: 6 in, 1 out]
  n385 = call <vilib>:"8_16_matrix_vector_multiply.vi"() -> ()  [unwired: 6 in, 1 out]
  n386 = call <vilib>:"8_15_matrix_vector_multiply.vi"() -> ()  [unwired: 6 in, 1 out]
  n387 = call <vilib>:"8_14_matrix_vector_multiply.vi"() -> ()  [unwired: 6 in, 1 out]
  n388 = call <vilib>:"8_13_matrix_vector_multiply.vi"() -> ()  [unwired: 6 in, 1 out]
  n389 = call <vilib>:"8_12_matrix_vector_multiply.vi"() -> ()  [unwired: 6 in, 1 out]
  n390 = call <vilib>:"8_11_matrix_vector_multiply.vi"() -> ()  [unwired: 6 in, 1 out]
  n391 = call <vilib>:"8_10_matrix_vector_multiply.vi"() -> ()  [unwired: 6 in, 1 out]
  n392 = call <vilib>:"8_9_matrix_vector_multiply.vi"() -> ()  [unwired: 6 in, 1 out]
  n393 = call <vilib>:"8_8_matrix_vector_multiply.vi"() -> ()  [unwired: 6 in, 1 out]
  n394 = call <vilib>:"8_7_matrix_vector_multiply.vi"() -> ()  [unwired: 6 in, 1 out]
  n395 = call <vilib>:"8_6_matrix_vector_multiply.vi"() -> ()  [unwired: 6 in, 1 out]
  n396 = call <vilib>:"8_5_matrix_vector_multiply.vi"() -> ()  [unwired: 6 in, 1 out]
  n397 = call <vilib>:"8_4_matrix_vector_multiply.vi"() -> ()  [unwired: 6 in, 1 out]
  n398 = call <vilib>:"8_3_matrix_vector_multiply.vi"() -> ()  [unwired: 6 in, 1 out]
  n399 = call <vilib>:"8_2_matrix_vector_multiply.vi"() -> ()  [unwired: 6 in, 1 out]
  n400 = call <vilib>:"8_1_matrix_vector_multiply.vi"() -> ()  [unwired: 6 in, 1 out]
  n401 = call <vilib>:"7_16_matrix_vector_multiply.vi"() -> ()  [unwired: 6 in, 1 out]
  n402 = call <vilib>:"7_15_matrix_vector_multiply.vi"() -> ()  [unwired: 6 in, 1 out]
  n403 = call <vilib>:"7_14_matrix_vector_multiply.vi"() -> ()  [unwired: 6 in, 1 out]
  n404 = call <vilib>:"7_13_matrix_vector_multiply.vi"() -> ()  [unwired: 6 in, 1 out]
  n405 = call <vilib>:"7_12_matrix_vector_multiply.vi"() -> ()  [unwired: 6 in, 1 out]
  n406 = call <vilib>:"7_11_matrix_vector_multiply.vi"() -> ()  [unwired: 6 in, 1 out]
  n407 = call <vilib>:"7_10_matrix_vector_multiply.vi"() -> ()  [unwired: 6 in, 1 out]
  n408 = call <vilib>:"7_9_matrix_vector_multiply.vi"() -> ()  [unwired: 6 in, 1 out]
  n409 = call <vilib>:"7_8_matrix_vector_multiply.vi"() -> ()  [unwired: 6 in, 1 out]
  n410 = call <vilib>:"7_7_matrix_vector_multiply.vi"() -> ()  [unwired: 6 in, 1 out]
  n411 = call <vilib>:"7_6_matrix_vector_multiply.vi"() -> ()  [unwired: 6 in, 1 out]
  n412 = call <vilib>:"7_5_matrix_vector_multiply.vi"() -> ()  [unwired: 6 in, 1 out]
  n413 = call <vilib>:"7_4_matrix_vector_multiply.vi"() -> ()  [unwired: 6 in, 1 out]
  n414 = call <vilib>:"7_3_matrix_vector_multiply.vi"() -> ()  [unwired: 6 in, 1 out]
  n415 = call <vilib>:"7_2_matrix_vector_multiply.vi"() -> ()  [unwired: 6 in, 1 out]
  n416 = call <vilib>:"7_1_matrix_vector_multiply.vi"() -> ()  [unwired: 6 in, 1 out]
  n417 = call <vilib>:"6_16_matrix_vector_multiply.vi"() -> ()  [unwired: 6 in, 1 out]
  n418 = call <vilib>:"6_15_matrix_vector_multiply.vi"() -> ()  [unwired: 6 in, 1 out]
  n419 = call <vilib>:"6_14_matrix_vector_multiply.vi"() -> ()  [unwired: 6 in, 1 out]
  n420 = call <vilib>:"6_13_matrix_vector_multiply.vi"() -> ()  [unwired: 6 in, 1 out]
  n421 = call <vilib>:"6_12_matrix_vector_multiply.vi"() -> ()  [unwired: 6 in, 1 out]
  n422 = call <vilib>:"6_11_matrix_vector_multiply.vi"() -> ()  [unwired: 6 in, 1 out]
  n423 = call <vilib>:"6_10_matrix_vector_multiply.vi"() -> ()  [unwired: 6 in, 1 out]
  n424 = call <vilib>:"6_9_matrix_vector_multiply.vi"() -> ()  [unwired: 6 in, 1 out]
  n425 = call <vilib>:"6_8_matrix_vector_multiply.vi"() -> ()  [unwired: 6 in, 1 out]
  n426 = call <vilib>:"6_7_matrix_vector_multiply.vi"() -> ()  [unwired: 6 in, 1 out]
  n427 = call <vilib>:"6_6_matrix_vector_multiply.vi"() -> ()  [unwired: 6 in, 1 out]
  n428 = call <vilib>:"6_5_matrix_vector_multiply.vi"() -> ()  [unwired: 6 in, 1 out]
  n429 = call <vilib>:"6_4_matrix_vector_multiply.vi"() -> ()  [unwired: 6 in, 1 out]
  n430 = call <vilib>:"6_3_matrix_vector_multiply.vi"() -> ()  [unwired: 6 in, 1 out]
  n431 = call <vilib>:"6_2_matrix_vector_multiply.vi"() -> ()  [unwired: 6 in, 1 out]
  n432 = call <vilib>:"6_1_matrix_vector_multiply.vi"() -> ()  [unwired: 6 in, 1 out]
  n433 = call <vilib>:"5_16_matrix_vector_multiply.vi"() -> ()  [unwired: 6 in, 1 out]
  n434 = call <vilib>:"5_15_matrix_vector_multiply.vi"() -> ()  [unwired: 6 in, 1 out]
  n435 = call <vilib>:"5_14_matrix_vector_multiply.vi"() -> ()  [unwired: 6 in, 1 out]
  n436 = call <vilib>:"5_13_matrix_vector_multiply.vi"() -> ()  [unwired: 6 in, 1 out]
  n437 = call <vilib>:"5_12_matrix_vector_multiply.vi"() -> ()  [unwired: 6 in, 1 out]
  n438 = call <vilib>:"5_11_matrix_vector_multiply.vi"() -> ()  [unwired: 6 in, 1 out]
  n439 = call <vilib>:"5_10_matrix_vector_multiply.vi"() -> ()  [unwired: 6 in, 1 out]
  n440 = call <vilib>:"5_9_matrix_vector_multiply.vi"() -> ()  [unwired: 6 in, 1 out]
  n441 = call <vilib>:"5_8_matrix_vector_multiply.vi"() -> ()  [unwired: 6 in, 1 out]
  n442 = call <vilib>:"5_7_matrix_vector_multiply.vi"() -> ()  [unwired: 6 in, 1 out]
  n443 = call <vilib>:"5_6_matrix_vector_multiply.vi"() -> ()  [unwired: 6 in, 1 out]
  n444 = call <vilib>:"5_5_matrix_vector_multiply.vi"() -> ()  [unwired: 6 in, 1 out]
  n445 = call <vilib>:"5_4_matrix_vector_multiply.vi"() -> ()  [unwired: 6 in, 1 out]
  n446 = call <vilib>:"5_3_matrix_vector_multiply.vi"() -> ()  [unwired: 6 in, 1 out]
  n447 = call <vilib>:"5_2_matrix_vector_multiply.vi"() -> ()  [unwired: 6 in, 1 out]
  n448 = call <vilib>:"5_1_matrix_vector_multiply.vi"() -> ()  [unwired: 6 in, 1 out]
  n449 = call <vilib>:"4_16_matrix_vector_multiply.vi"() -> ()  [unwired: 6 in, 1 out]
  n450 = call <vilib>:"4_15_matrix_vector_multiply.vi"() -> ()  [unwired: 6 in, 1 out]
  n451 = call <vilib>:"4_14_matrix_vector_multiply.vi"() -> ()  [unwired: 6 in, 1 out]
  n452 = call <vilib>:"4_13_matrix_vector_multiply.vi"() -> ()  [unwired: 6 in, 1 out]
  n453 = call <vilib>:"4_12_matrix_vector_multiply.vi"() -> ()  [unwired: 6 in, 1 out]
  n454 = call <vilib>:"4_11_matrix_vector_multiply.vi"() -> ()  [unwired: 6 in, 1 out]
  n455 = call <vilib>:"4_10_matrix_vector_multiply.vi"() -> ()  [unwired: 6 in, 1 out]
  n456 = call <vilib>:"4_9_matrix_vector_multiply.vi"() -> ()  [unwired: 6 in, 1 out]
  n457 = call <vilib>:"4_8_matrix_vector_multiply.vi"() -> ()  [unwired: 6 in, 1 out]
  n458 = call <vilib>:"4_7_matrix_vector_multiply.vi"() -> ()  [unwired: 6 in, 1 out]
  n459 = call <vilib>:"4_6_matrix_vector_multiply.vi"() -> ()  [unwired: 6 in, 1 out]
  n460 = call <vilib>:"4_5_matrix_vector_multiply.vi"() -> ()  [unwired: 6 in, 1 out]
  n461 = call <vilib>:"4_4_matrix_vector_multiply.vi"() -> ()  [unwired: 6 in, 1 out]
  n462 = call <vilib>:"4_3_matrix_vector_multiply.vi"() -> ()  [unwired: 6 in, 1 out]
  n463 = call <vilib>:"4_2_matrix_vector_multiply.vi"() -> ()  [unwired: 6 in, 1 out]
  n464 = call <vilib>:"4_1_matrix_vector_multiply.vi"() -> ()  [unwired: 6 in, 1 out]
  n465 = call <vilib>:"3_16_matrix_vector_multiply.vi"() -> ()  [unwired: 6 in, 1 out]
  n466 = call <vilib>:"3_15_matrix_vector_multiply.vi"() -> ()  [unwired: 6 in, 1 out]
  n467 = call <vilib>:"3_14_matrix_vector_multiply.vi"() -> ()  [unwired: 6 in, 1 out]
  n468 = call <vilib>:"3_13_matrix_vector_multiply.vi"() -> ()  [unwired: 6 in, 1 out]
  n469 = call <vilib>:"3_12_matrix_vector_multiply.vi"() -> ()  [unwired: 6 in, 1 out]
  n470 = call <vilib>:"3_11_matrix_vector_multiply.vi"() -> ()  [unwired: 6 in, 1 out]
  n471 = call <vilib>:"3_10_matrix_vector_multiply.vi"() -> ()  [unwired: 6 in, 1 out]
  n472 = call <vilib>:"3_9_matrix_vector_multiply.vi"() -> ()  [unwired: 6 in, 1 out]
  n473 = call <vilib>:"3_8_matrix_vector_multiply.vi"() -> ()  [unwired: 6 in, 1 out]
  n474 = call <vilib>:"3_7_matrix_vector_multiply.vi"() -> ()  [unwired: 6 in, 1 out]
  n475 = call <vilib>:"3_6_matrix_vector_multiply.vi"() -> ()  [unwired: 6 in, 1 out]
  n476 = call <vilib>:"3_5_matrix_vector_multiply.vi"() -> ()  [unwired: 6 in, 1 out]
  n477 = call <vilib>:"3_4_matrix_vector_multiply.vi"() -> ()  [unwired: 6 in, 1 out]
  n478 = call <vilib>:"3_3_matrix_vector_multiply.vi"() -> ()  [unwired: 6 in, 1 out]
  n479 = call <vilib>:"3_2_matrix_vector_multiply.vi"() -> ()  [unwired: 6 in, 1 out]
  n480 = call <vilib>:"3_1_matrix_vector_multiply.vi"() -> ()  [unwired: 6 in, 1 out]
  n481 = call <vilib>:"2_16_matrix_vector_multiply.vi"() -> ()  [unwired: 6 in, 1 out]
  n482 = call <vilib>:"2_15_matrix_vector_multiply.vi"() -> ()  [unwired: 6 in, 1 out]
  n483 = call <vilib>:"2_14_matrix_vector_multiply.vi"() -> ()  [unwired: 6 in, 1 out]
  n484 = call <vilib>:"2_13_matrix_vector_multiply.vi"() -> ()  [unwired: 6 in, 1 out]
  n485 = call <vilib>:"2_12_matrix_vector_multiply.vi"() -> ()  [unwired: 6 in, 1 out]
  n486 = call <vilib>:"2_11_matrix_vector_multiply.vi"() -> ()  [unwired: 6 in, 1 out]
  n487 = call <vilib>:"2_10_matrix_vector_multiply.vi"() -> ()  [unwired: 6 in, 1 out]
  n488 = call <vilib>:"2_9_matrix_vector_multiply.vi"() -> ()  [unwired: 6 in, 1 out]
  n489 = call <vilib>:"2_8_matrix_vector_multiply.vi"() -> ()  [unwired: 6 in, 1 out]
  n490 = call <vilib>:"2_7_matrix_vector_multiply.vi"() -> ()  [unwired: 6 in, 1 out]
  n491 = call <vilib>:"2_6_matrix_vector_multiply.vi"() -> ()  [unwired: 6 in, 1 out]
  n492 = call <vilib>:"2_5_matrix_vector_multiply.vi"() -> ()  [unwired: 6 in, 1 out]
  n493 = call <vilib>:"2_4_matrix_vector_multiply.vi"() -> ()  [unwired: 6 in, 1 out]
  n494 = call <vilib>:"2_3_matrix_vector_multiply.vi"() -> ()  [unwired: 6 in, 1 out]
  n495 = call <vilib>:"2_2_matrix_vector_multiply.vi"() -> ()  [unwired: 6 in, 1 out]
  n496 = call <vilib>:"2_1_matrix_vector_multiply.vi"() -> ()  [unwired: 6 in, 1 out]
  n497 = call <vilib>:"1_16_matrix_vector_multiply.vi"() -> ()  [unwired: 6 in, 1 out]
  n498 = call <vilib>:"1_15_matrix_vector_multiply.vi"() -> ()  [unwired: 6 in, 1 out]
  n499 = call <vilib>:"1_14_matrix_vector_multiply.vi"() -> ()  [unwired: 6 in, 1 out]
  n500 = call <vilib>:"1_13_matrix_vector_multiply.vi"() -> ()  [unwired: 6 in, 1 out]
  n501 = call <vilib>:"1_12_matrix_vector_multiply.vi"() -> ()  [unwired: 6 in, 1 out]
  n502 = call <vilib>:"1_11_matrix_vector_multiply.vi"() -> ()  [unwired: 6 in, 1 out]
  n503 = call <vilib>:"1_10_matrix_vector_multiply.vi"() -> ()  [unwired: 6 in, 1 out]
  n504 = call <vilib>:"1_9_matrix_vector_multiply.vi"() -> ()  [unwired: 6 in, 1 out]
  n505 = call <vilib>:"1_8_matrix_vector_multiply.vi"() -> ()  [unwired: 6 in, 1 out]
  n506 = call <vilib>:"1_7_matrix_vector_multiply.vi"() -> ()  [unwired: 6 in, 1 out]
  n507 = call <vilib>:"1_6_matrix_vector_multiply.vi"() -> ()  [unwired: 6 in, 1 out]
  n508 = call <vilib>:"1_5_matrix_vector_multiply.vi"() -> ()  [unwired: 6 in, 1 out]
  n509 = call <vilib>:"1_4_matrix_vector_multiply.vi"() -> ()  [unwired: 6 in, 1 out]
  n510 = call <vilib>:"1_3_matrix_vector_multiply.vi"() -> ()  [unwired: 6 in, 1 out]
  n511 = call <vilib>:"1_2_matrix_vector_multiply.vi"() -> ()  [unwired: 6 in, 1 out]
  n512 = call <vilib>:"1_1_matrix_vector_multiply.vi"() -> ()  [unwired: 6 in, 1 out]
  n513 = call <vilib>:"matrix_vector_multiply_SGL.vi"() -> ()  [unwired: 6 in, 1 out]
